vi "APC_9049_u162float.vi"(1 "min":sgl[](array[numeric]), 2 "holding register values":u16[](array[numeric]), 3 "max":sgl[](array[numeric])) -> (0 "Array":sgl[](array[numeric]))   [LabVIEW 2020]
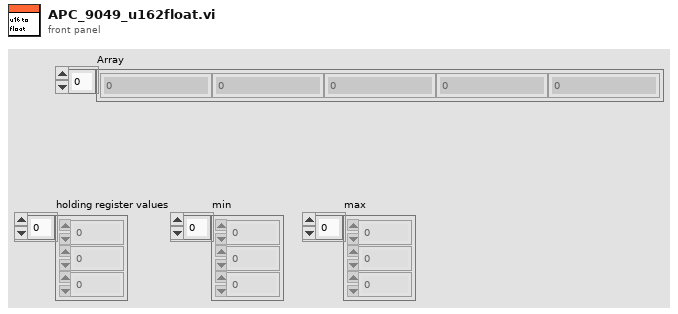
[diagram p1: front panel]
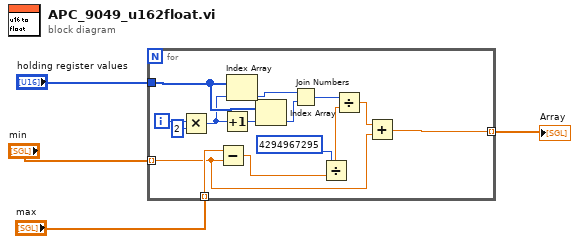
[diagram p0: block diagram]
diagram:
  n1 = for {
    tunnel: "holding register values" -> [w15]
    tunnel: "min" -> [w6] mode=indexing
    tunnel: "max" -> [w18] mode=indexing
    tunnel: [w5] -> w1 mode=indexing
    i -> [w17]
    n2 = Multiply(x=w17, y=2) -> (x*y=w13:i32)
    n3 = Subtract(x=w18, y=w6) -> (x-y=w10:sgl)
    n4 = Increment(x=w13) -> (x+1=w14:i32)
    n5 = Index Array(array=w15, index=w13) -> (element=w12:u16)
    n6 = Index Array(array=w15, index=w14) -> (element=w11:u16)
    n7 = Join Numbers(hi=w12, lo=w11) -> ((hi.lo)=w9:u32)
    n8 = Divide(x=u32 4294967295, y=w10) -> (x/y=w8:sgl)
    n9 = Divide(x=w9, y=w8) -> (x/y=w7:sgl)
    n10 = Add(x=w7, y=w6) -> (x+y=w5:sgl)
  }
  "Array" <- w1
